vi "Close.vi"(8 "error in (no error)":errorcluster, 11 "Modbus instance in":refnum<class "Modbus API.lvclass">) -> (0 "error out":errorcluster)   [LabVIEW 2020, in "SubVIs.lvlib" / "Modbus API.lvclass"]
doc: "Performs any actions needed to shutdown and clean up the Modbus instance provided."
uses:
  <vilib>/Modbus/subvis/Modbus API/Modbus API.lvclass
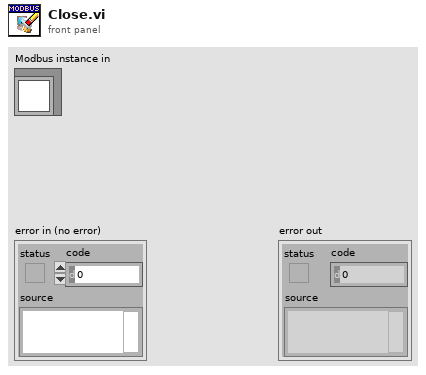
[diagram p1: front panel]
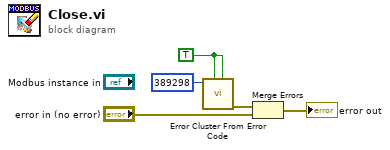
[diagram p0: block diagram]
diagram:
  w1 = TRUE ("show call chain? (False)")
  n1 = call <vilib>:"Error Cluster From Error Code.vi"("is warning? (False)"=w1, "show call chain? (False)"=w1, "error code (0)"=389298) -> ("error out"=w3:errorcluster)  [unwired: 6 in]
  n2 = Merge Errors(w3, "error in (no error)") -> (→"error out":errorcluster)
